vi "Target Heater Table Filename (Read).vi"(6 "ISOBUS address":T5=-1 caption="ISOBUS address (-1)", 8 "error in":errorcluster, 11 "Mercury Reference In":T2) -> (0 "error out":errorcluster, 2 "Target Heater Table Filename":string, 3 "Mercury Reference Out":T2, 4 "Valid?":T1)   [LabVIEW 2018, in "Mercury iXX.lvlib" / "Control Loop.lvlib"]
doc: "Read the filename of the target heater table."
uses:
  Control Loop.lvlib
  Mercury Reference.ctl
  Comms Transport Layer.ctl
  Query Dynamic Reference.ctl
  ISOBus Address.ctl
  Is Valid LED.ctl
  Command Verbs.ctl
  Mercury iXX.lvlib
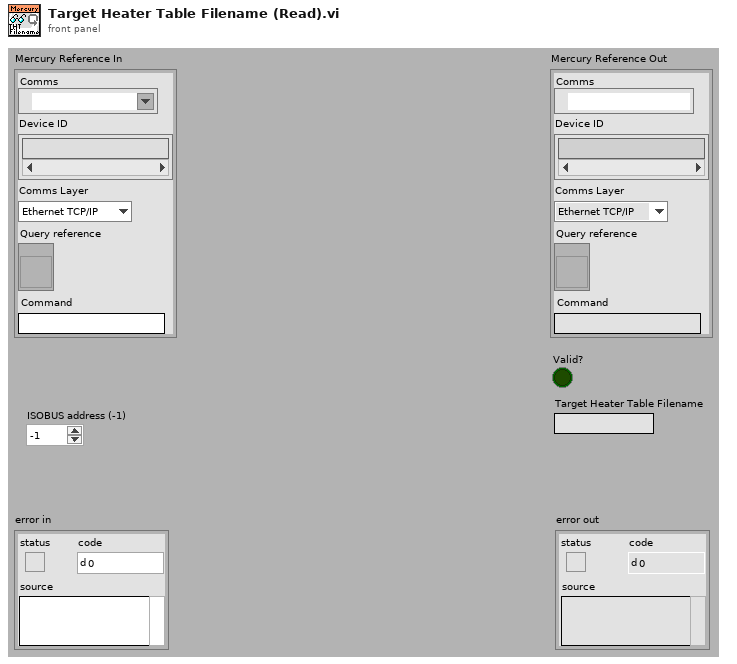
[diagram p1: front panel]
types:
  T1 = typedef "Mercury iXX.lvlib/Is Valid LED.ctl" = bool
  T2 = typedef "Mercury iXX.lvlib/Mercury Reference.ctl" = cluster{"Comms":refnum<visa-resource-name>, "Device ID":string[], "Comms Layer":T3, "Command":string, "Query reference":T4}
  T3 = typedef "Mercury iXX.lvlib/Comms Transport Layer.ctl" = enum16{"Ethernet TCP/IP", "USB", "ISOBus - RS-232", "GPIB"}
  T4 = typedef "Mercury iXX.lvlib/Query Dynamic Reference.ctl" = refnum<vi>
  T5 = typedef "Mercury iXX.lvlib/ISOBus Address.ctl" = i32
  T6 = typedef "Mercury iXX.lvlib/Command Verbs.ctl" = string
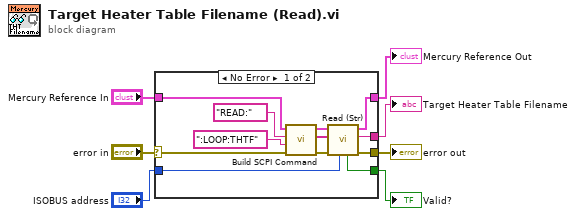
[diagram p0: block diagram]
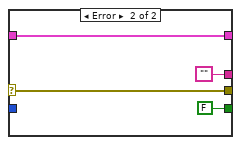
[diagram p2: hidden frame]
diagram:
  n1 = case shown="No Error" "error in" {
    selector: "error in" -> [w13 w22]
    tunnel: "Mercury Reference In" -> [w14 w23]
    tunnel: [w8 w23] -> w4
    tunnel: [w11 w22] -> w1
    tunnel: "ISOBUS address" -> [w12 _]
    tunnel: [w9 ""] -> w3
    tunnel: [w10 FALSE ("Valid?")] -> w2
    frame No Error {
      n2 = call "Build SCPI Command.vi"("error in"=w13, "Noun(s)"=":LOOP:THTF" ("Command"), "Verb"=T6 "READ:", "Mercury Reference In"=w14) -> ("error out"=w15:errorcluster, "SCPI Message(s)"=w18:string[], "Mercury Reference Out"=w17:T2)  [unwired: 5 out]
      n3 = call "Read (Str).vi"("ISOBUS address"=w12, "error in"=w15, "SCPI Message(s)"=w18, "Mercury Reference In"=w17) -> ("error out"=w11:errorcluster, "Response"=w9:string, "Mercury Reference Out"=w8:T2, "Valid?"=w10:T1)  [unwired: 4 out]
    }
    frame Error {
    }
  }
  "Mercury Reference Out" <- w4
  "Target Heater Table Filename" <- w3
  "error out" <- w1
  "Valid?" <- w2
